vi "SeCrTs-NS Reader.vi"(8 "error in":errorcluster, 9 "Err":refnum<queue>, 10 "Data":refnum<notifier>, 11 "Message Queues in":T1) -> (0 "error out":errorcluster, 2 "Available Elements for Reading":i32)   [LabVIEW 2022 SP3]
uses:
  UI Message handler/Message Queue/Message Queue.lvlib
  <resource>/objmgr/ni.dex.rc
  Controls/SeCrTs-NS Data type.ctl
  UI Message handler/Message Queue/Message Cluster.ctl
  UI Message handler/Message Queue/All Message Queues.ctl
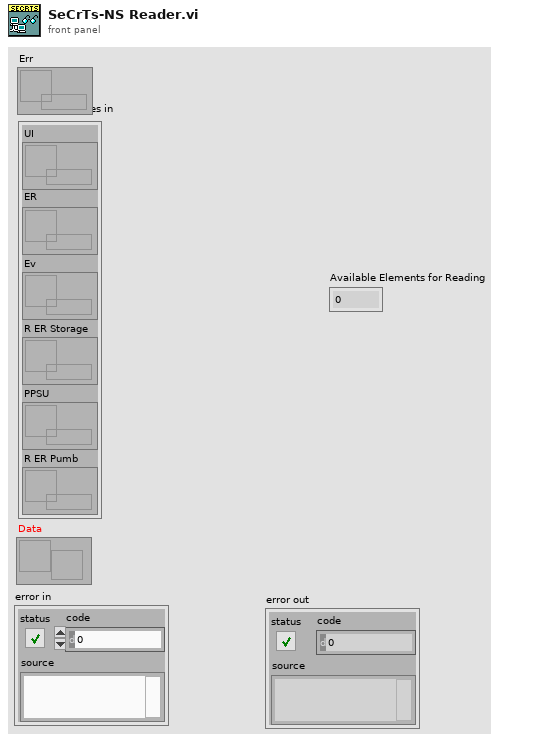
[diagram p1: front panel]
types:
  T1 = typedef "Message Queue.lvlib/All Message Queues.ctl" = cluster{"UI":refnum<queue>, "ER":refnum<queue>, "Ev":refnum<queue>, "R ER Storage":refnum<queue>, "PPSU":refnum<queue>, "R ER Pumb":refnum<queue>}
  T2 = cluster{"Error Code":string, "Error Source":string}
  T3 = typedef "NS Data type.ctl" = cluster{"DI_Data":digitalwaveform[], "Drive_A_C":waveform(dbl)[], "Drive_A_D":waveform(dbl)[], "Drive_L_C":waveform(dbl)[], "Drive_L_D":waveform(dbl)[], "Loop Status":bool[], "CDT":dbl, "RT Error":cluster{"Error Code":string, "Error Source":string}, "DO":waveform(dbl)[], "SEQ Monitor":string[]}
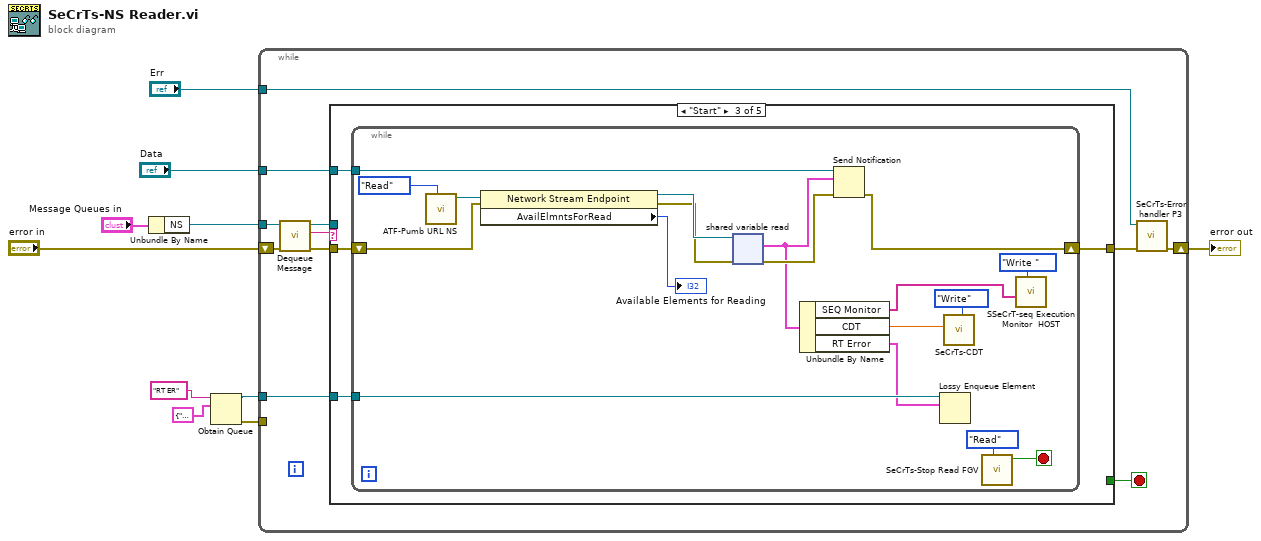
[diagram p0: block diagram]
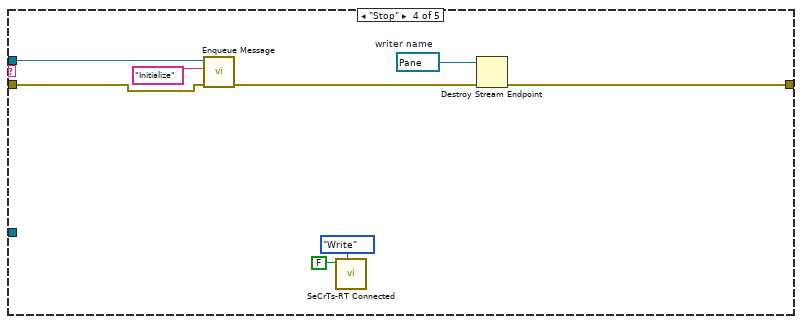
[diagram p4: hidden frame]
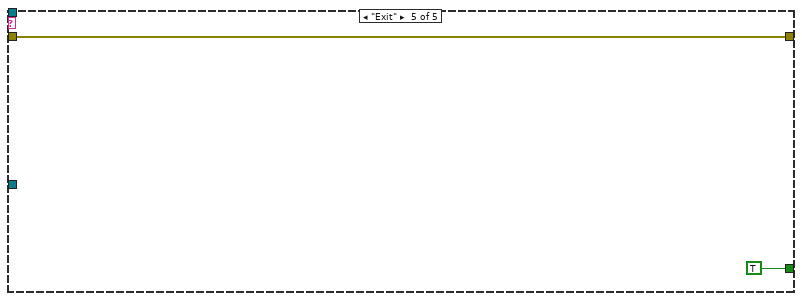
[diagram p5: hidden frame]
diagram:
  n1 = Unbundle By Name("Message Queues in") -> ("NS"=w9:refnum<queue>)
  n2 = Obtain Queue(name (unnamed)="RT ER", element data type=T2 {"Error Code"="", "Error Source"=""} ("RT Error")) -> (queue out=w3:refnum<queue>, error out=w2:errorcluster)  [unwired: 3 in, 1 out]
  n3 = while {
    tunnel: w9 -> [w18]
    shift-right: [w13] -> w8
    shift-left: "error in" -> [w19]
    tunnel: "Data" -> [w15]
    tunnel: "Err" -> [w12]
    tunnel: w3 -> [w11]
    tunnel: w2 -> [_]
    stop <- w21 stop-if-true
    n4 = call "Dequeue Message.vi"("error in (no error)"=w19, "Message Queue"=w18) -> ("error out"=w16:errorcluster, "Message"=w20:string, "dup Message Queue"=w17:refnum<queue>)  [unwired: 6 in, 1 out]
    n5 = case shown="\"Start\"" w20 {
      tunnel: [_ _ _ _ TRUE] -> w21
      tunnel: w17 -> [_ _ _ w53 _]
      tunnel: w16 -> [w22 w23 w27 w51 w54]
      tunnel: [w22 w23 w25 w49 w54] -> w14
      tunnel: w15 -> [_ _ w26 _ _]
      tunnel: w11 -> [_ _ w24 _ _]
      frame Default {
      }
      frame "Initialize" {
      }
      frame "Start" {
        n6 = while {
          tunnel: w26 -> [w44]
          shift-right: [w43] -> w25
          shift-left: w27 -> [w45]
          tunnel: w24 -> [w33]
          stop <- w34 stop-if-true
          n7 = call "ATF-Pumb URL NS.vi"("Enum"=enum16{"Init", "Read", "Write"}."Read") -> ("Pumb writer  2"=w36:refnum<k21>)  [unwired: 9 in, 1 out]
          n8 = property class="Network Stream Endpoint"(reference=w36, error in=w45) -> (reference out=w42:refnum<k21>, error out=w41:errorcluster, "AvailElmntsForRead"=→"Available Elements for Reading":i32)
          n9 = shared-variable-read(w42, w41) -> (w40:errorcluster, w38:T3)  [unwired: 1 in, 2 out]
          n10 = Unbundle By Name(w38) -> ("SEQ Monitor"=w29:string[], "CDT"=w32:dbl, "RT Error"=w30:T2)
          n11 = Send Notification(notification=w38, notifier=w44, error in (no error)=w40) -> (error out=w43:errorcluster)  [unwired: 1 out]
          n12 = Lossy Enqueue Element(queue=w33, element=w30) -> ()  [unwired: 1 in, 4 out]
          n13 = call "SeCrTs-CDT.vi"("CDT"=w32, "Write/Read"=enum16{"Write", "Read"}."Write") -> ()  [unwired: 8 in, 2 out]
          n14 = call "SeCrTs-Stop Read FGV.vi"("Enum"=enum16{"Init", "Read", "Write"}."Read") -> ("Stop R"=w34:bool)  [unwired: 10 in]
          n15 = call "SSeCrT-seq Execution Monitor  HOST.vi"("Enum"=enum16{"Read", "Write "}."Write ", "Seq Monitor"=w29) -> ()  [unwired: 8 in, 2 out]
        }
      }
      frame "Stop" {
        w48 = refnum<k21> refnum  # writer name
        n16 = call "Enqueue Message.vi"("error in (no error)"=w51, "Message"="Initialize", "Message Queue"=w53) -> ("error out"=w50:errorcluster)  [unwired: 7 in, 1 out]
        n17 = call "SeCrTs-RT Connected .vi"("Enum"=enum16{"Read", "Write"}."Write", "Storage rt con"=FALSE ("rt con")) -> ()  [unwired: 7 in, 3 out]
        n18 = Destroy Stream Endpoint(8:w50, 11:w48) -> (0:w49:errorcluster)
      }
      frame "Exit" {
      }
    }
    n19 = call "SeCrTs-Error handler P3.vi"("error in"=w14, "Message Queue"=w12) -> ("error out"=w13:errorcluster)  [unwired: 8 in, 1 out]
  }
  "error out" <- w8
